vi "SIM Clear Node Execution.vi"(8 "error in (no error)":errorcluster, 11 "node ref":refnum<vi>) -> (0 "error out":errorcluster, 2 "succeeded":bool, 3 "dup node ref":refnum<vi>)   [LabVIEW 2017]
panel:
  # "Calling this VI will clear any configured Sim Node execution \nand cause the Node to execute on all steps including Minor \nTimesteps in Simulations configured with solvers other than \nRK1 (Euler) or Discrete States only."
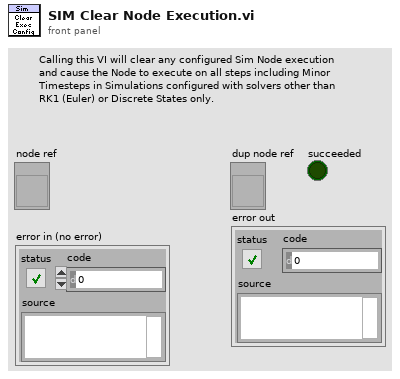
[diagram p1: front panel]
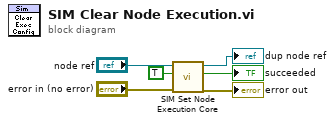
[diagram p0: block diagram]
diagram:
  n1 = call <vilib>:"SIM Set Node Execution Core.vi"("error in (no error)"="error in (no error)", "clear tag (f)"=TRUE, "Node in"="node ref") -> ("error out"=→"error out":errorcluster, "succeeded"=→"succeeded":bool, "Node out"=→"dup node ref":refnum<vi>)  [unwired: 6 in]
